vi "Execute Statement.vi"(6 "Values in":string[](array[string]), 8 "error in (no error)":errorcluster, 9 "Parameters in":string[](array[string]), 10 "Statement index in":u64, 11 "mysql in":refnum<class "mysql.lvclass">) -> (0 "error out":errorcluster, 2 "Result":string[][](array[string]), 3 "mysql out":refnum<class "mysql.lvclass">)   [LabVIEW 2020, in "mysql.lvlib" / "mysql.lvclass"]
uses:
  mysql.lvclass
  database-interface/IDatabase/IDatabase/IDatabase.lvclass
panel:
  # "Implementation may change this connector pane.\nThis is just a guess."
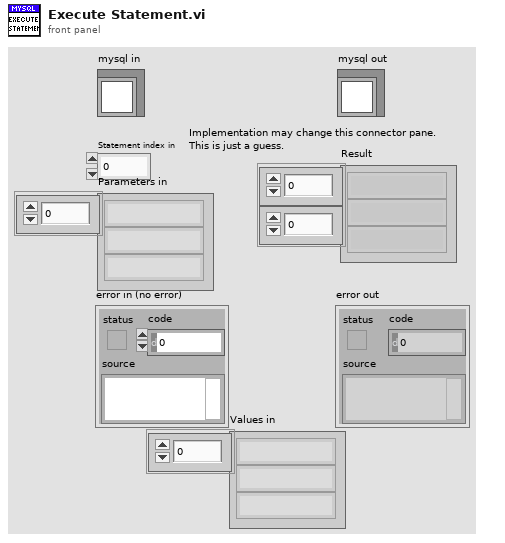
[diagram p1: front panel]
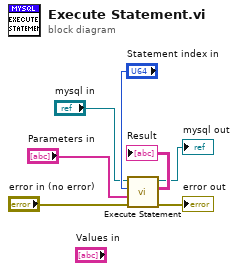
[diagram p0: block diagram]
diagram:
  n1 = call-parent "Execute Statement.vi"("error in (no error)"="error in (no error)", "Parameters in"="Parameters in", "Statement index in"="Statement index in", "IDatabase in"="mysql in") -> ("error out"=→"error out":errorcluster, "Result"=→"Result":string[][], "IDatabase out"=→"mysql out":refnum<class "mysql.lvclass">)  [unwired: 5 in]
